vi "action.vi"(0 "NInstrSim_ConfigureVDCRange":refnum<class "NInstrSim_ConfigureVDCRange.lvclass">, 2 "HGF_Visitable":refnum<class "HGF_Visitable.lvclass">, 5 "error in (no error)":errorcluster) -> (14 "dup NInstrSim_ConfigureVDCRange":refnum<class "NInstrSim_ConfigureVDCRange.lvclass">, 16 "dup HGF_Visitable":refnum<class "HGF_Visitable.lvclass">, 19 "error out":errorcluster)   [LabVIEW 2009, in "HB_Device_Examples.lvlib" / "NInstrSim_ConfigureVDCRange.lvclass"]
doc: "This is a dynamic dispatch VI that is called from Visitor.visit(). It will call member VIs of Visitable to perform the requested action which means: calling public methods of Visitable child class.\n\n<B>Hint:</B> This method is abstract and need to be implemented by child classes."
uses:
  NInstrSim_ConfigureVDCRange.lvclass
  lib.lib/HGF_LVC/HGF_BaseClasses/HGF_Visitable/HGF_Visitable.lvclass
  NInstrSim.lvclass
  NInstrSim_ConfigureVDCRange.lvclass/NInstrSim_ConfigureVDCRange.ctl
  lib.lib/HGF_LVC/HGF_BaseClasses/HGF_NetworkVisitor/HGF_NetworkVisitor.lvclass
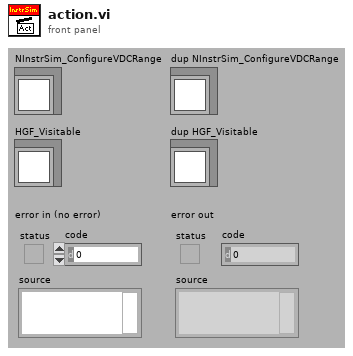
[diagram p1: front panel]
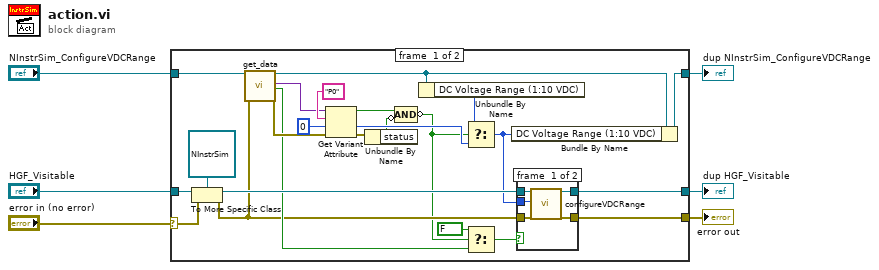
[diagram p0: block diagram]
diagram:
  n1 = case shown="No Error" "error in (no error)" {
    selector: "error in (no error)" -> [w25 w38]
    tunnel: "NInstrSim_ConfigureVDCRange" -> [w15 w40]
    tunnel: "HGF_Visitable" -> [w30 w39]
    tunnel: [w27 w39] -> w4
    tunnel: [w26 w38] -> w3
    tunnel: [w13 w40] -> w1
    frame #0 {
      n2 = To More Specific Class(target class=refnum<class "NInstrSim.lvclass"> refnum ("HB_HGF_Test.lvlib:NInstrSim.lvclass"), reference=w30, error in=w25) -> (specific class reference=w28:refnum<class "NInstrSim.lvclass">, error out=w19:errorcluster)
      n3 = call "get_data.vi"("HGF_NetworkData"=w15, "error in (no error)"=w19) -> ("dup HGF_NetworkData"=w14:refnum<class "NInstrSim_ConfigureVDCRange.lvclass">, "data"=w11:variant, "no link"=w20:bool, "error out"=w21:errorcluster)  [unwired: 14 out]
      n4 = Get Variant Attribute(Variant=w11, name="P0", default value (empty Variant)=u16 0 ("DC Voltage Range (1:10 VDC)"), error in=w21) -> (found=w9:bool, value=w22:u16, error out=w8:errorcluster)  [unwired: 1 out]
      n5 = Unbundle By Name(w8) -> ("status"=w10:bool)
      n6 = Compound Arithmetic op=AND(w9, invert w10) -> (invert w7:bool)
      n7 = Unbundle By Name(w14) -> ("DC Voltage Range (1:10 VDC)"=w18:u16)
      n8 = Select(t=w18, s=w7, f=w22) -> (s? t:f=w12:u16)
      n9 = Select(t=FALSE, s=w7, f=w20) -> (s? t:f=w16:bool)
      n10 = Bundle By Name(cluster=w14, "DC Voltage Range (1:10 VDC)"=w12) -> (w13:refnum<class "NInstrSim_ConfigureVDCRange.lvclass">)
      n11 = case shown="False" w16 {
        tunnel: w28 -> [w35 w37]
        tunnel: [w34 w37] -> w27
        tunnel: [w33 w36] -> w26
        tunnel: w19 -> [w32 w36]
        tunnel: w12 -> [w31 _]
        frame #0 {
          n12 = call "configureVDCRange.vi"("NInstrSim"=w35, "DC Voltage Range (1:10 VDC)"=w31, "error in (no error)"=w32) -> ("dup NInstrSim"=w34:refnum<class "NInstrSim.lvclass">, "error out"=w33:errorcluster)  [unwired: 15 out]
        }
        frame #1 {
        }
      }
    }
    frame #1 {
    }
  }
  "error out" <- w3
  "dup NInstrSim_ConfigureVDCRange" <- w1
  "dup HGF_Visitable" <- w4
